vi "5.vi"   [LabVIEW 2017, in "ErrorStructureDrawer-Tests.lvlib"]
uses:
  ErrorStructureDrawer-Tests.lvlib
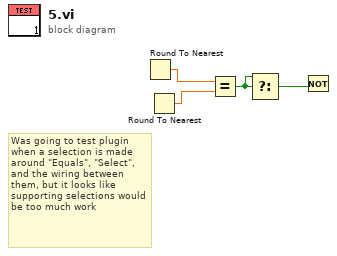
[diagram p0: block diagram]
diagram:
  # "Was going to test plugin when a selection is made around \"Equals\", \"Select\", and the wiring between them, but it looks like supporting selections would be too much work"
  n1 = Round To Nearest() -> (nearest integer value=w4:dbl)  [unwired: 1 in]
  n2 = Round To Nearest() -> (nearest integer value=w3:dbl)  [unwired: 1 in]
  n3 = Equal?(x=w4, y=w3) -> (x = y?=w2:bool)
  n4 = Select(t=w2, s=w2) -> (s? t:f=w1:bool)  [unwired: 1 in]
  n5 = Not(x=w1) -> ()  [unwired: 1 out]
